vi "retrieveNewData.vi"(8 "error in (no error)":errorcluster, 10 "model":refnum<class "Model.lvclass">, 11 "SamplingState in":refnum<class "SamplingState.lvclass">) -> (0 "error out":errorcluster, 2 "model 2":refnum<class "Model.lvclass">, 3 "SamplingState out":refnum<class "SamplingState.lvclass">)   [LabVIEW 2013, in "SamplingState.lvclass"]
uses:
  SamplingState.lvclass
  Model/Model/Model.lvclass
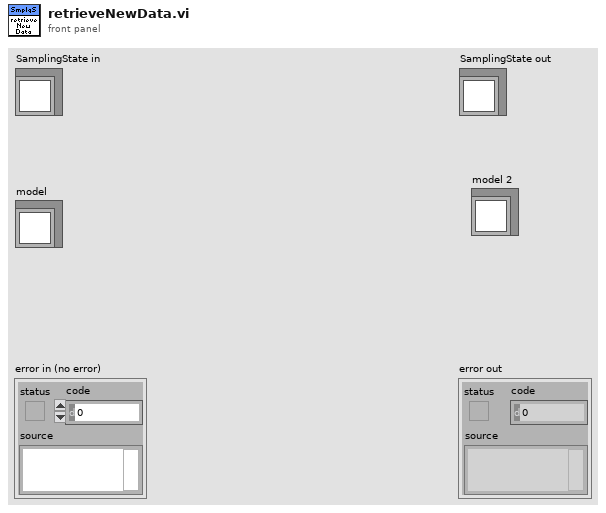
[diagram p1: front panel]
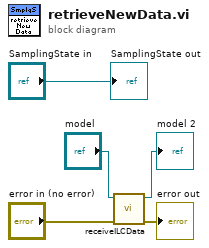
[diagram p0: block diagram]
diagram:
  n1 = call "receiveILCData.vi"("error in (no error)"="error in (no error)", "Model in"="model") -> ("error out"=→"error out":errorcluster, "Model out"=→"model 2":refnum<class "Model.lvclass">)  [unwired: 8 in]
  "SamplingState out" <- "SamplingState in"
